vi "Numeric Assert.vi"() -> ()   [LabVIEW 2016]
uses:
  Core/AssertEngine/AssertEngine.lvlib
panel:
  in  "Top Level VI Name":string
  in  "Assert VI UID":i32
  in  "Calling VI Name":string
  in  "Comment":string
  in  "Assert VI Name":string
  in  "Default Failure Action":string
  in  "Assert Builder":string
  in  "Build Timestamp":timestamp
  in  "Eval String":string
  in  "Passed?":bool
  in  "Assert Name":string
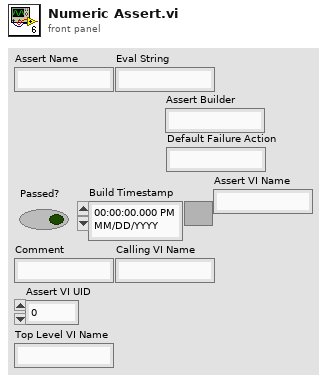
[diagram p1: front panel]
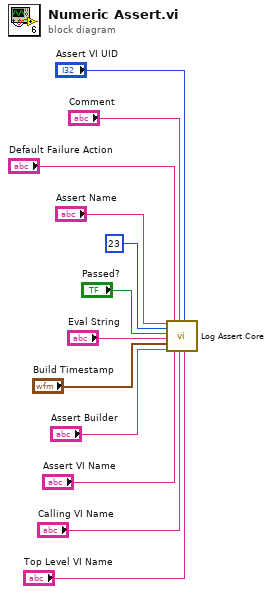
[diagram p0: block diagram]
diagram:
  n1 = call "Log Assert Core.vi"("Assert Name"="Assert Name", "Data Value"=23, "Passed?"="Passed?", "Eval String"="Eval String", "Build Timestamp"="Build Timestamp", "Assert Builder"="Assert Builder", "Default Failure Action"="Default Failure Action", "Assert VI Name"="Assert VI Name", "Comment"="Comment", "Calling VI Name"="Calling VI Name", "Assert VI UID"="Assert VI UID", "Top Level VI Name"="Top Level VI Name") -> ()  [unwired: 8 in]
